vi "Run VI.vi"(2 "error in (no error)":errorcluster caption="错误输入（无错误）", 3 "VI Reference in":refnum<vi>) -> (0 "error out":errorcluster caption="错误输出", 1 "VI Reference out":refnum<vi>)   [LabVIEW 2016]
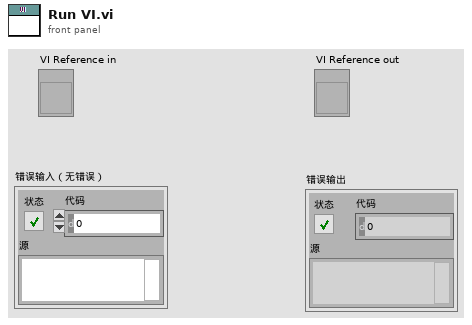
[diagram p1: front panel]
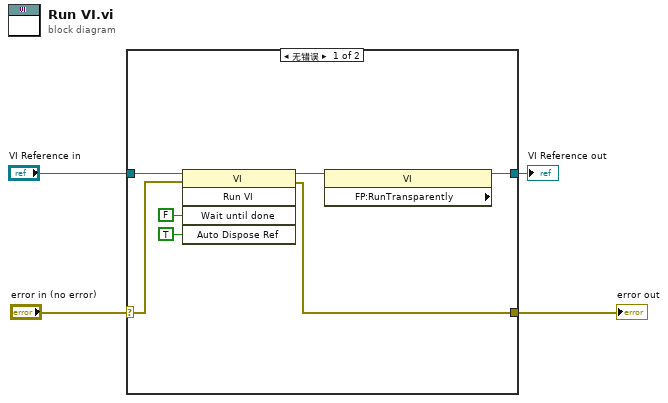
[diagram p0: block diagram]
diagram:
  n1 = case shown="无错误" "error in (no error)" {
    selector: "error in (no error)" -> [w8 w13]
    tunnel: "VI Reference in" -> [w9 w12]
    tunnel: [w7 w13] -> w2
    tunnel: [w5 w12] -> w1
    frame No Error {
      n2 = invoke class="VI" method="Run VI"(reference=w9, error in=w8, "Wait until done"=FALSE ("结束前等待"), "Auto Dispose Ref"=TRUE ("自动销毁引用")) -> (reference out=w6:refnum<vi>, error out=w7:errorcluster)  [unwired: 1 in, 3 out]
      n3 = property class="VI" props=["FP:RunTransparently"](reference=w6) -> (reference out=w5:refnum<vi>)  [unwired: 1 in, 2 out]
    }
    frame Error {
    }
  }
  "error out" <- w2
  "VI Reference out" <- w1
